vi "Configure Output.vi"(8 "error in":errorcluster, 11 "FGen PXI Base CFG in":refnum<class "FGen PXI Base CFG.lvclass">) -> (0 "error out":errorcluster, 3 "FGen PXI Base CFG out":refnum<class "FGen PXI Base CFG.lvclass">)   [LabVIEW 2023, in "FGen PXI Base CFG.lvlib" / "FGen PXI Base CFG.lvclass"]
uses:
  FGen PXI Base CFG.lvclass
  FGen PXI Base CFG.lvclass/FGen PXI Base CFG.ctl
  Configuration/Configuration JSON/Configuration JSON Base/CFG JSON.lvclass/CFG JSON.ctl
  7d5647a1-ee57-477e-af02-dfb71140fe97.vi
  <vilib>/JDP Science/JSONtext/Find Item.vi
  <vilib>/JDP Science/JSONtext/Next JSON Value.vi
  <vilib>/JDP Science/JSONtext/String Subset.vi
  <vilib>/JDP Science/JSONtext/Parsing/Advance past next JSON Value (inlined COPY).vi
  <vilib>/JDP Science/JSONtext/Parsing/Advance past whitespace.vi
  <vilib>/JDP Science/JSONtext/Parsing/Advance past String.vi
  <vilib>/JDP Science/JSONtext/Parsing/Advance past Number.vi
  <vilib>/JDP Science/JSONtext/Parsing/Advance past Line Ending.vi
  <vilib>/JDP Science/JSONtext/Parsing/Parse Full Path or Item Name.vi
  <vilib>/JDP Science/JSONtext/Parsing/Advance past Array.vi
  <vilib>/JDP Science/JSONtext/Parsing/Advance past Object.vi
  <vilib>/JDP Science/JSONtext/support/Error Cluster From Code.vi
  <vilib>/JDP Science/JSONtext/Offset/Find Item Locations by Path.vi
  <vilib>/JDP Science/JSONtext/JSON text to Variant.vi
  <vilib>/Utility/error.llb/Error Cluster From Error Code.vi
  <vilib>/JDP Science/JSONtext/LVClass Serializer/JSONtext LVClass Serializer.lvclass
  <vilib>/ErrorRing/Error Ring.xnode
  Configuration/Configuration JSON/Configuration JSON Base/CFG JSON.lvclass
  D:/git/HAL/HAL GOOP4/FGen/FGen Base CFG/FGen Base CFG.lvclass
  D:/git/HAL/HAL GOOP4/Configuration/Configuration JSON/Configuration JSON Base/CFG JSON.lvclass
  D:/git/HAL/HAL GOOP4/Interfaces/IConfigure/IConfigure.lvclass
  D:/git/HAL/HAL GOOP4/FGen/FGen PXI/FGen PXI Base CFG/FGen PXI Base CFG.lvclass
panel:
  out "Advanced:Idle Behavior":i32(ring)=400 items=["Hold Last Value"=400, "Jump To Value"=401]
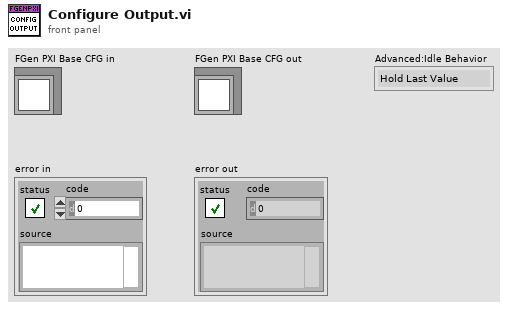
[diagram p1: front panel]
types:
  T1 = cluster{"Idle Behavior":string, "Idle Value":i32, "Digital Gain":dbl}
  T2 = typedef "LVStringsAndValuesArrayTypeDef_I32.ctl" = cluster{"String":string, "Value":i32}[]
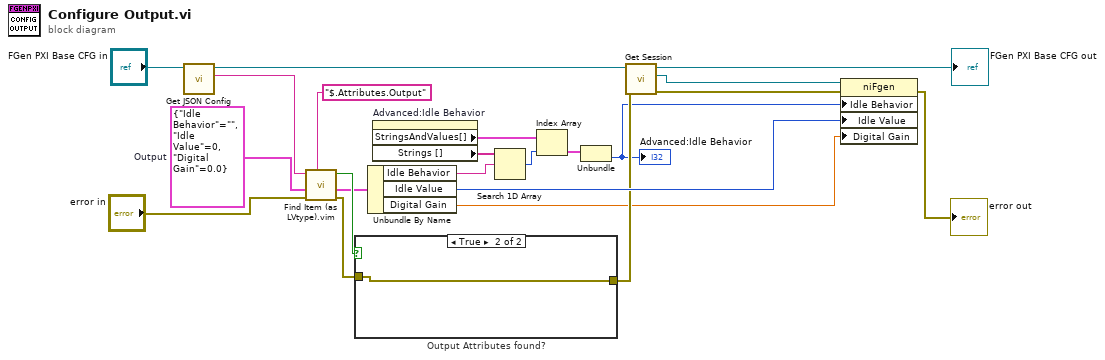
[diagram p0: block diagram]
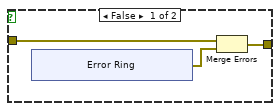
[diagram p2: hidden frame]
diagram:
  w16 = T1 {"Idle Behavior"="", "Idle Value"=0, "Digital Gain"=0.0}  # Output
  n1 = call "Get JSON Config.vi"("CFG Base in"="FGen PXI Base CFG in") -> ("<JSON>Config>"=w17:string, "CFG Base out"=w18:refnum<class "FGen PXI Base CFG.lvclass">)  [unwired: 9 in]
  n2 = call "Find Item (as LVtype).vim"("$Path or Item Name"="$.Attributes.Output", "error in (no error)"="error in", "Data Type and Default Value"=w16, "JSON"=w17) -> ("error out"=w14:errorcluster, "Data"=w13:T1, "Found"=w15:bool)  [unwired: 4 in, 1 out]
  n3 = case "Output Attributes found?" shown="True" w15 {
    tunnel: w14 -> [w25 w31]
    tunnel: [w23 w31] -> w7
    frame False {
      n4 = xnode "Error Ring"() -> ("error out"=w24:errorcluster)
      n5 = Merge Errors(w25, w24) -> (w23:errorcluster)
    }
    frame True {
    }
  }
  n6 = Unbundle By Name(w13) -> ("Idle Behavior"=w12:string, "Idle Value"=w8:i32, "Digital Gain"=w2:dbl)
  n7 = property on="Advanced:Idle Behavior" class="Ring (strict)"() -> ("StringsAndValues[]"=w11:T2, "Strings []"=w20:string[])  [unwired: 2 in, 2 out]
  n8 = Search 1D Array(1D array=w20, element=w12) -> (index of element=w6:i32)  [unwired: 1 in]
  n9 = Index Array(array=w11, index=w6) -> (element=w10:cluster{"String":string, "Value":i32})
  n10 = Unbundle(w10) -> ("Value"=w4:i32)  [unwired: 1 out]
  "Advanced:Idle Behavior" <- w4
  n11 = call "Get Session.vi"("error in (no error)"=w7, "FGen PXI Base CFG in"=w18) -> ("error out"=w9:errorcluster, "Session"=w21:refnum<k15>, "FGen PXI Base CFG out"=→"FGen PXI Base CFG out":refnum<class "FGen PXI Base CFG.lvclass">)  [unwired: 7 in]
  n12 = property class="niFgen"(reference=w21, error in=w9, "Idle Behavior"=w4, "Idle Value"=w8, "Digital Gain"=w2) -> (error out=→"error out":errorcluster)  [unwired: 1 out]
